vi "PathPlanner_ConstraintsZone_OverlapsRange.vi"(9 "MaxPos":dbl, 10 "MinPos":dbl, 11 "ConstraintsZone":T1) -> (3 "OverlapsRange":bool)   [LabVIEW 2019, in "PathPlanner24.lvlib"]
doc: "Get if this zone overlaps a given range\n\nInputs:\n -- ConstraintsZone - cluster - zone definition. \n -- minPos - double - The minimum waypoint relative position of the range\n -- maxPos - double - The maximum waypoint relative position of the range\n\nOutputs:\n -- OverlapsRange - boolean - True if any part of this zone is within the given range"
uses:
  PathPlanner24.lvlib
  TypeDef/PathPlannerConstraintsZone.ctl
  TypeDef/PathPlannerPathConstraints.ctl
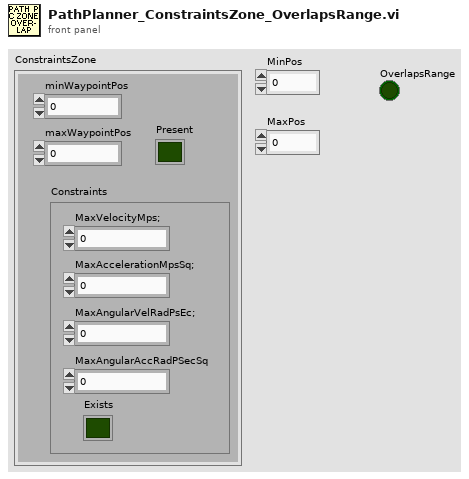
[diagram p1: front panel]
types:
  T1 = typedef "PathPlanner24.lvlib/PathPlannerConstraintsZone.ctl" = cluster{"minWaypointPos":dbl, "maxWaypointPos":dbl, "Constraints":T2, "Present":bool}
  T2 = typedef "PathPlanner24.lvlib/PathPlannerPathConstraints.ctl" = cluster{"MaxVelocityMps;":dbl, "MaxAccelerationMpsSq;":dbl, "MaxAngularVelRadPsEc;":dbl, "MaxAngularAccRadPSecSq":dbl, "Exists":bool}
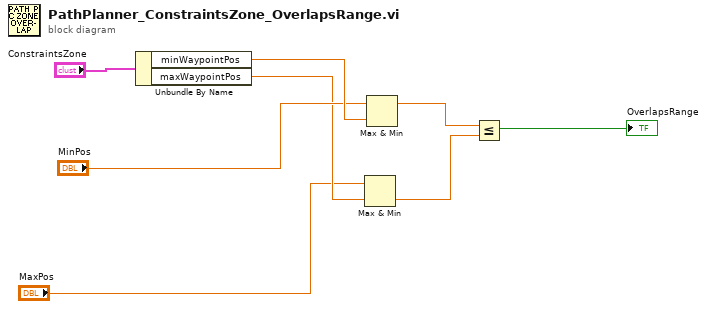
[diagram p0: block diagram]
diagram:
  n1 = Unbundle By Name("ConstraintsZone") -> ("minWaypointPos"=w7:dbl, "maxWaypointPos"=w4:dbl)
  n2 = Max & Min(x="MaxPos", y=w4) -> (min(x,y)=w2:dbl)  [unwired: 1 out]
  n3 = Max & Min(x="MinPos", y=w7) -> (max(x,y)=w5:dbl)  [unwired: 1 out]
  n4 = Less Or Equal?(x=w5, y=w2) -> (x <= y?=→"OverlapsRange":bool)
